vi "write_xively.vi"(1 "Solar__Tilted_":dbl, 2 "Solar__Tracked_":dbl, 3 "Solar__Vertical_":dbl, 4 "Solar__meteo_":dbl, 5 "Thin_Film_2":dbl, 6 "Thin_Film_1":dbl, 7 "Poly Si":dbl, 8 "Poly Si":dbl, 9 "DSSC3":dbl, 10 "DSSC2":dbl, 11 "DSSC1":dbl) -> ()   [LabVIEW 2012]
uses:
  <vilib>/httpClient/LabVIEWHTTPClient.lvlib
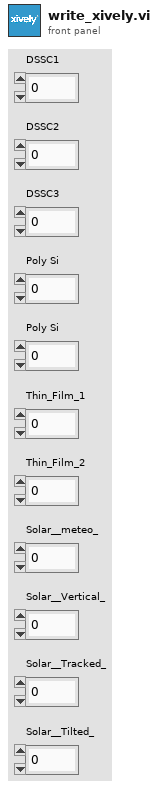
[diagram p1: front panel]
types:
  T1 = typedef "LabVIEWHTTPClient.lvlib/ClientHandle.ctl" = refnum<k1>
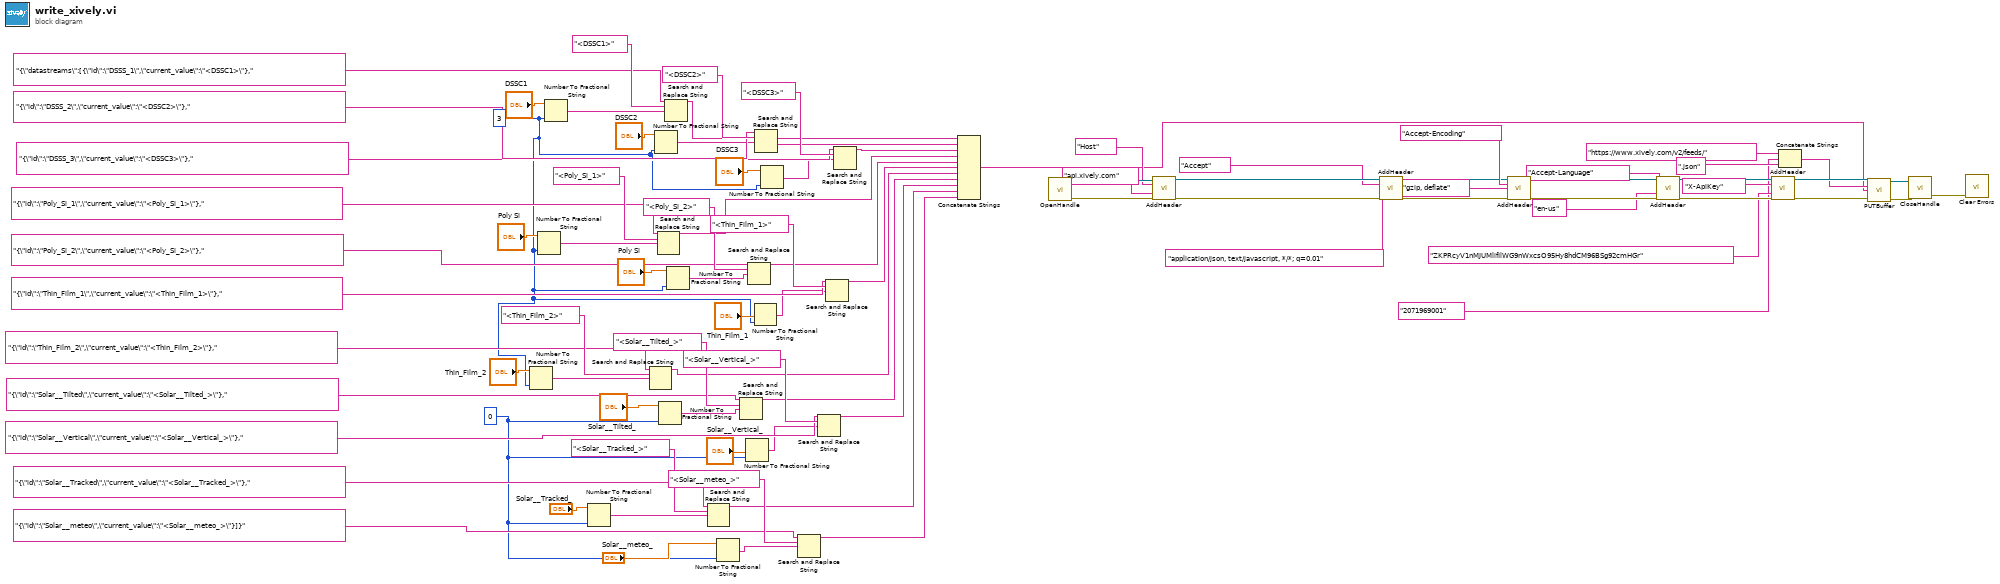
[diagram p0: block diagram]
diagram:
  w1 = i16 0 ("precision (6)")
  w2 = i16 3 ("precision (6)")
  n1 = Number To Fractional String(number="Thin_Film_2", precision (6)=w2) -> (F-format string=w42:string)  [unwired: 2 in]
  n2 = Number To Fractional String(number="Poly Si", precision (6)=w2) -> (F-format string=w49:string)  [unwired: 2 in]
  n3 = Number To Fractional String(number="DSSC1", precision (6)=w2) -> (F-format string=w64:string)  [unwired: 2 in]
  n4 = Number To Fractional String(number="Solar__Tracked_", precision (6)=w1) -> (F-format string=w35:string)  [unwired: 2 in]
  n5 = Search and Replace String(input string="{\"id\":\"Thin_Film_2\",\"current_value\":\"<Thin_Film_2>\"},", search string="<Thin_Film_2>", replace string=w42) -> (result string=w19:string)  [unwired: 5 in, 3 out]
  n6 = Number To Fractional String(number="DSSC2", precision (6)=w2) -> (F-format string=w30:string)  [unwired: 2 in]
  n7 = Search and Replace String(input string="{\"id\":\"Poly_Si_1\",\"current_value\":\"<Poly_Si_1>\"},", search string="<Poly_Si_1>", replace string=w49) -> (result string=w26:string)  [unwired: 5 in, 3 out]
  n8 = Number To Fractional String(number="Solar__Tilted_", precision (6)=w1) -> (F-format string=w21:string)  [unwired: 2 in]
  n9 = Search and Replace String(input string="{\"datastreams\":[{\"id\":\"DSSS_1\",\"current_value\":\"<DSSC1>\"},", search string="<DSSC1>", replace string=w64) -> (result string=w6:string)  [unwired: 5 in, 3 out]
  n10 = Number To Fractional String(number="Poly Si", precision (6)=w2) -> (F-format string=w22:string)  [unwired: 2 in]
  n11 = Search and Replace String(input string="{\"id\":\"Solar__Tracked\",\"current_value\":\"<Solar__Tracked_>\"},", search string="<Solar__Tracked_>", replace string=w35) -> (result string=w16:string)  [unwired: 5 in, 3 out]
  n12 = Number To Fractional String(number="Solar__meteo_", precision (6)=w1) -> (F-format string=w8:string)  [unwired: 2 in]
  n13 = Search and Replace String(input string="{\"id\":\"Solar__Tilted\",\"current_value\":\"<Solar__Tilted_>\"},", search string="<Solar__Tilted_>", replace string=w21) -> (result string=w18:string)  [unwired: 5 in, 3 out]
  n14 = Number To Fractional String(number="Solar__Vertical_", precision (6)=w1) -> (F-format string=w20:string)  [unwired: 2 in]
  n15 = Search and Replace String(input string="{\"id\":\"Poly_Si_2\",\"current_value\":\"<Poly_Si_2>\"},", search string="<Poly_Si_2>", replace string=w22) -> (result string=w25:string)  [unwired: 5 in, 3 out]
  n16 = Number To Fractional String(number="Thin_Film_1", precision (6)=w2) -> (F-format string=w23:string)  [unwired: 2 in]
  n17 = Search and Replace String(input string="{\"id\":\"DSSS_2\",\"current_value\":\"<DSSC2>\"},", search string="<DSSC2>", replace string=w30) -> (result string=w52:string)  [unwired: 5 in, 3 out]
  n18 = Number To Fractional String(number="DSSC3", precision (6)=w2) -> (F-format string=w29:string)  [unwired: 2 in]
  n19 = Search and Replace String(input string="{\"id\":\"Solar__meteo\",\"current_value\":\"<Solar__meteo_>\"}]}", search string="<Solar__meteo_>", replace string=w8) -> (result string=w5:string)  [unwired: 5 in, 3 out]
  n20 = Search and Replace String(input string="{\"id\":\"Solar__Vertical\",\"current_value\":\"<Solar__Vertical_>\"},", search string="<Solar__Vertical_>", replace string=w20) -> (result string=w17:string)  [unwired: 5 in, 3 out]
  n21 = Search and Replace String(input string="{\"id\":\"Thin_Film_1\",\"current_value\":\"<Thin_Film_1>\"},", search string="<Thin_Film_1>", replace string=w23) -> (result string=w24:string)  [unwired: 5 in, 3 out]
  n22 = Search and Replace String(input string="{\"id\":\"DSSS_3\",\"current_value\":\"<DSSC3>\"},", search string="<DSSC3>", replace string=w29) -> (result string=w51:string)  [unwired: 5 in, 3 out]
  n23 = Concatenate Strings(w6, w52, w51, w26, w25, w24, w19, w18, w17, w16, w5) -> (w4:string)
  n24 = call <vilib>:"OpenHandle.vi"() -> ("client handle out"=w83:T1, "error out"=w82:errorcluster)  [unwired: 14 in]
  n25 = call <vilib>:"AddHeader.vi"("client handle"=w83, "header"="Host", "value"="api.xively.com", "error in (no error)"=w82) -> ("client handle out"=w79:T1, "error out"=w78:errorcluster)  [unwired: 10 in]
  n26 = call <vilib>:"AddHeader.vi"("client handle"=w79, "header"="Accept", "value"="application/json, text/javascript, */*; q=0.01", "error in (no error)"=w78) -> ("client handle out"=w74:T1, "error out"=w73:errorcluster)  [unwired: 10 in]
  n27 = call <vilib>:"AddHeader.vi"("client handle"=w74, "header"="Accept-Encoding", "value"="gzip, deflate", "error in (no error)"=w73) -> ("client handle out"=w71:T1, "error out"=w70:errorcluster)  [unwired: 10 in]
  n28 = call <vilib>:"AddHeader.vi"("client handle"=w71, "header"="Accept-Language", "value"="en-us", "error in (no error)"=w70) -> ("client handle out"=w67:T1, "error out"=w66:errorcluster)  [unwired: 10 in]
  n29 = call <vilib>:"AddHeader.vi"("client handle"=w67, "header"="X-ApiKey", "value"="ZKPRcyV1nMJUMlifIlWG9nWxcsO95Hy8hdCM96BSg92cmHGr" ("API Key"), "error in (no error)"=w66) -> ("client handle out"=w86:T1, "error out"=w85:errorcluster)  [unwired: 10 in]
  n30 = Concatenate Strings("https://www.xively.com/v2/feeds/" ("url"), "2071969001" ("Feed ID"), ".json" ("string")) -> (w61:string)
  n31 = call <vilib>:"PUTBuffer.vi"("client handle"=w86, "url"=w61, "buffer"=w4, "error in (no error)"=w85) -> ("client handle out"=w60:T1, "error out"=w59:errorcluster)  [unwired: 8 in, 2 out]
  n32 = call <vilib>:"CloseHandle.vi"("client handle"=w60, "error in (no error)"=w59) -> ("error out"=w3:errorcluster)  [unwired: 13 in]
  n33 = call <vilib>:"Clear Errors.vi"("error in (no error)"=w3) -> ()  [unwired: 6 in, 1 out]
